vi "Enable Lighting Read.vi"(8 "error in (no error)":errorcluster, 11 "3D Plot.lvclass in":refnum<class "3D Plot.lvclass">) -> (0 "error out":errorcluster, 1 "Enable Lighting?":bool, 3 "3D Plot.lvclass out":refnum<class "3D Plot.lvclass">)   [LabVIEW 2017, in "3D Plot.lvclass"]
uses:
  <vilib>/Math Plots/3D Math Plots/3D Plot/3D Plot/3D Plot.lvclass
  <vilib>/Math Plots/3D Math Plots/3D Plot/3D Plot/3D Plot.lvclass/3D Plot.ctl
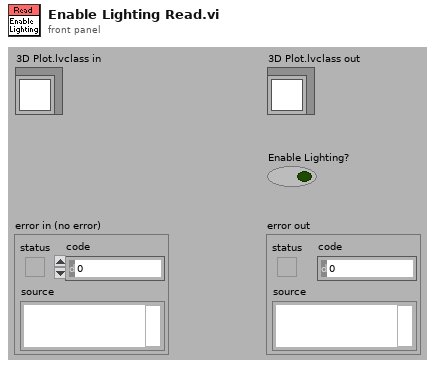
[diagram p1: front panel]
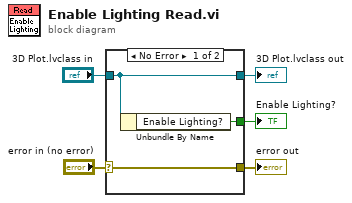
[diagram p0: block diagram]
diagram:
  n1 = case shown="No Error" "error in (no error)" {
    selector: "error in (no error)" -> [w7 w9]
    tunnel: [w8 _] -> w5
    tunnel: "3D Plot.lvclass in" -> [w6 w10]
    tunnel: [w7 w9] -> w2
    tunnel: [w6 w10] -> w1
    frame No Error {
      n2 = Unbundle By Name(w6) -> ("Enable Lighting?"=w8:bool)
    }
    frame Error {
    }
  }
  "Enable Lighting?" <- w5
  "error out" <- w2
  "3D Plot.lvclass out" <- w1
